vi "DSF.Engine.Transceiver Thread.Transfer.Build.vi"(8 "error in (no error)":errorcluster, 10 "Transfer":refnum<class "DSF.Engine.Transfer.lvclass">, 11 "Transceiver Thread in":refnum<class "DSF.Engine.Transceiver Thread.lvclass">) -> (0 "error out":errorcluster, 3 "Transceiver Thread out":refnum<class "DSF.Engine.Transceiver Thread.lvclass">)   [LabVIEW 2017, in "DSF.Engine.lvlib" / "DSF.Engine.Transceiver Thread.lvclass"]
uses:
  DSF.Engine.Transceiver Thread.lvclass
  Buffer/DSF.Engine.Memory.Buffer.lvclass
  Transfer/DSF.Engine.Transfer.lvclass
  Pointer/DSF.Engine.Pointer.DBL.lvclass
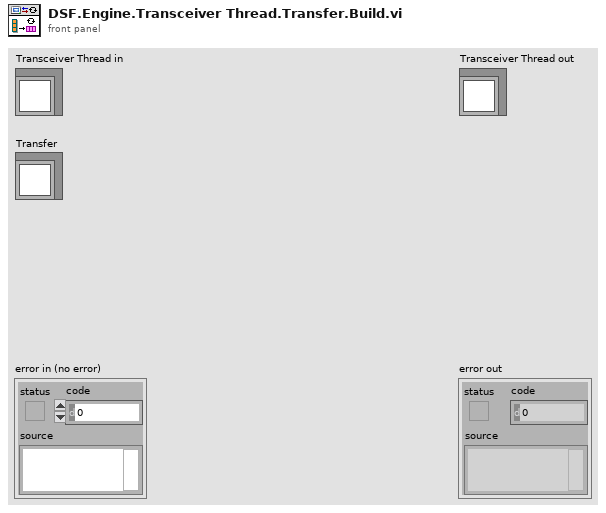
[diagram p1: front panel]
types:
  T1 = typedef "DSF.Shared.lvlib/DSF.Shared.Typedefs.Configuration.Transfer.Channel Block Descriptor.ctl" = cluster{"First Channel Descriptor":T2, "count":u64, "channel array index":u64}
  T2 = typedef "DSF.Shared.lvlib/DSF.Shared.Typedefs.Configuration.Transfer.Channel Descriptor.ctl" = cluster{"Channel Parameters":T3, "base address":u64}
  T3 = typedef "DSF.Shared.lvlib/DSF.Shared.Typedefs.Configuration.Transfer.Channel Parameters.ctl" = cluster{"offset":u64, "data type":T4}
  T4 = typedef "DSF.Shared.lvlib/DSF.Shared.Typedefs.Data Type.ctl" = enum8{"Bool", "SGL", "DBL", "I8", "I16", "I32", "I64", "U8", "U16", "U32", "U64"}
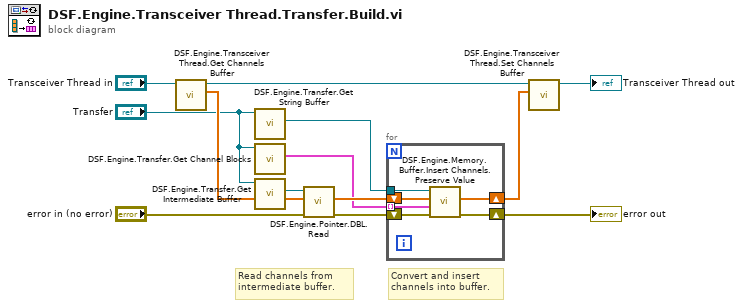
[diagram p0: block diagram]
diagram:
  # "Convert and insert channels into buffer."
  # "Read channels from intermediate buffer."
  n1 = call "DSF.Engine.Transceiver Thread.Get Channels Buffer.vi"("Transceiver Thread in"="Transceiver Thread in") -> ("channels buffer"=w6:dbl[], "Transceiver Thread out"=w4:refnum<class "DSF.Engine.Transceiver Thread.lvclass">)  [unwired: 9 in]
  n2 = call "DSF.Engine.Transfer.Get String Buffer.vi"("Transfer in"="Transfer") -> ("Buffer"=w12:refnum<class "DSF.Engine.Memory.Buffer.lvclass">)  [unwired: 9 in, 1 out]
  n3 = call "DSF.Engine.Transfer.Get Channel Blocks.vi"("Transfer in"="Transfer") -> ("Channel Blocks"=w1:T1[])  [unwired: 9 in, 1 out]
  n4 = call "DSF.Engine.Transfer.Get Intermediate Buffer.vi"("Transfer in"="Transfer") -> ("DBL Buffer"=w11:refnum<class "DSF.Engine.Pointer.DBL.lvclass">)  [unwired: 9 in, 1 out]
  n5 = call "DSF.Engine.Pointer.DBL.Read.vi"("error in (no error)"="error in (no error)", "buffer in"=w6, "DBL Pointer in"=w11) -> ("error out"=w8:errorcluster, "buffer out"=w9:dbl[])  [unwired: 6 in, 1 out]
  n6 = for {
    shift-right: [w17] -> w5
    shift-left: w9 -> [w18]
    shift-right: [w16] -> w13
    shift-left: w8 -> [w19]
    tunnel: w12 -> [w15]
    tunnel: w1 -> [w14] mode=indexing
    n7 = call "DSF.Engine.Memory.Buffer.Insert Channels.Preserve Value.vi"("error in (no error)"=w19, "channel block"=w14, "channels buffer in"=w18, "Buffer in"=w15) -> ("error out"=w16:errorcluster, "channels buffer out"=w17:dbl[])  [unwired: 5 in, 1 out]
  }
  "error out" <- w13
  n8 = call "DSF.Engine.Transceiver Thread.Set Channels Buffer.vi"("channels buffer"=w5, "Transceiver Thread in"=w4) -> ("Transceiver Thread out"=→"Transceiver Thread out":refnum<class "DSF.Engine.Transceiver Thread.lvclass">)  [unwired: 9 in]
